vi "Decision(SubVI).vi"(0 "L_ind0":i32, 1 "L_ind1":i32, 2 "Peak_ind0":dbl[](array[numeric]), 3 "Peak_ind1":dbl[](array[numeric])) -> (5 "L_sum":i32, 7 "Bits":dbl[](array[numeric]))   [LabVIEW 2017]
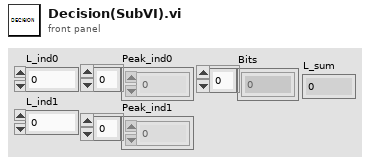
[diagram p1: front panel]
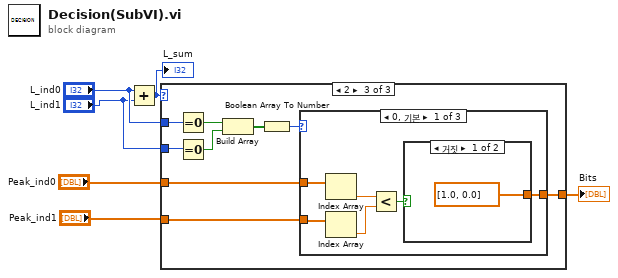
[diagram p0: block diagram]
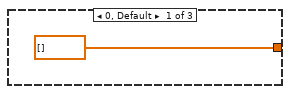
[diagram p2: hidden frame]
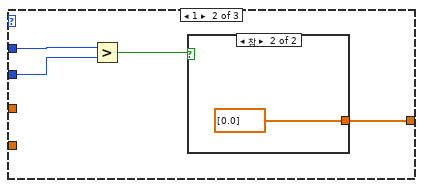
[diagram p3: hidden frame]
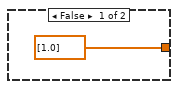
[diagram p4: hidden frame]
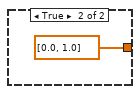
[diagram p5: hidden frame]
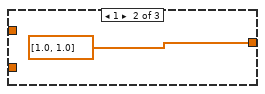
[diagram p6: hidden frame]
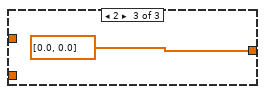
[diagram p7: hidden frame]
diagram:
  n1 = Add(x="L_ind0", y="L_ind1") -> (x+y=w3:i32)
  "L_sum" <- w3
  n2 = case shown="2" w3 {
    tunnel: [dbl[] [] w10 w16] -> w4
    tunnel: "L_ind0" -> [_ w9 w22]
    tunnel: "L_ind1" -> [_ w8 w21]
    tunnel: "Peak_ind0" -> [_ _ w15]
    tunnel: "Peak_ind1" -> [_ _ w14]
    frame 0, Default {
    }
    frame 1 {
      n3 = Greater?(x=w9, y=w8) -> (0:w11:bool)
      n4 = case shown="참" w11 {
        tunnel: [dbl[] [1.0] dbl[] [0.0]] -> w10
        frame False {
        }
        frame True {
        }
      }
    }
    frame 2 {
      n5 = Equal To 0?(x=w22) -> (x = 0?=w20:bool)
      n6 = Equal To 0?(x=w21) -> (x = 0?=w19:bool)
      n7 = Build Array(w20, w19) -> (w18:bool[])
      n8 = Boolean Array To Number(Boolean array=w18) -> (number=w17:u32)
      n9 = case shown="0, 기본" w17 {
        tunnel: [w23 dbl[] [1.0, 1.0] dbl[] [0.0, 0.0]] -> w16
        tunnel: w15 -> [w28 _ _]
        tunnel: w14 -> [w27 _ _]
        frame 0, Default {
          n10 = Index Array(array=w28) -> (element=w26:dbl)  [unwired: 1 in]
          n11 = Index Array(array=w27) -> (element=w25:dbl)  [unwired: 1 in]
          n12 = Less?(x=w26, y=w25) -> (x < y?=w24:bool)
          n13 = case shown="거짓" w24 {
            tunnel: [dbl[] [1.0, 0.0] dbl[] [0.0, 1.0]] -> w23
            frame False {
            }
            frame True {
            }
          }
        }
        frame 1 {
        }
        frame 2 {
        }
      }
    }
  }
  "Bits" <- w4
